vi "Find Control Index in Cluster.vi"(8 "error in (no error)":errorcluster, 10 "Control Name":string, 11 "Cluster ref in":refnum<vi>) -> (0 "error out":errorcluster, 2 "Control Index":i32, 3 "Cluster ref out":refnum<vi>)   [LabVIEW 2019, in "gRPC Template Creation Utility.lvlib"]
uses:
  gRPC Template Creation Utility.lvlib
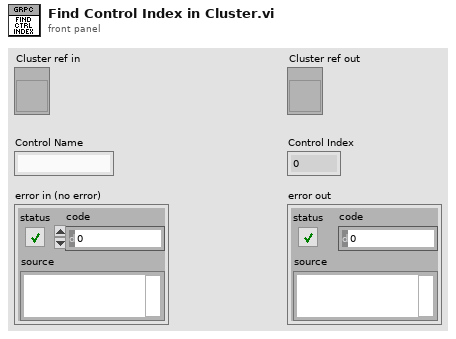
[diagram p1: front panel]
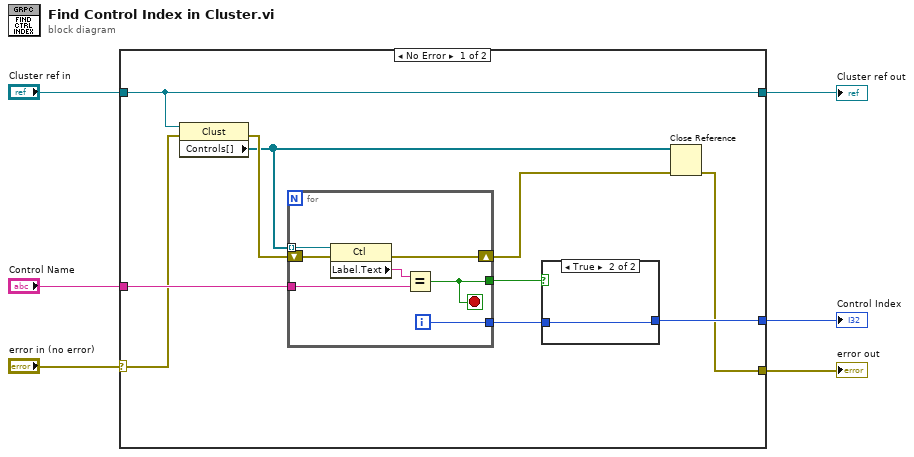
[diagram p0: block diagram]
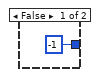
[diagram p2: hidden frame]
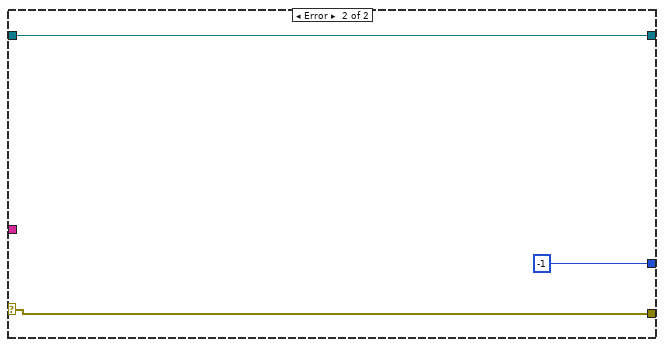
[diagram p3: hidden frame]
diagram:
  n1 = case shown="No Error" "error in (no error)" {
    selector: "error in (no error)" -> [w8 w27]
    tunnel: "Control Name" -> [w11 _]
    tunnel: "Cluster ref in" -> [w7 w26]
    tunnel: [w10 -1] -> w4
    tunnel: [w9 w27] -> w3
    tunnel: [w7 w26] -> w1
    frame No Error {
      n2 = property class="Clust"(reference=w7, error in=w8) -> (error out=w15:errorcluster, "Controls[]"=w14:refnum<vi>[])  [unwired: 1 out]
      n3 = for {
        tunnel: w14 -> [w25] mode=indexing
        tunnel: w11 -> [w24]
        tunnel: [w23] -> w12
        tunnel: [w22] -> w13
        shift-right: [w21] -> w16
        shift-left: w15 -> [w20]
        i -> [w22]
        stop <- w23 stop-if-true
        n4 = property class="Ctl"(reference=w25, error in=w20) -> (error out=w21:errorcluster, "Label.Text"=w19:string)  [unwired: 1 out]
        n5 = Equal?(x=w19, y=w24) -> (x = y?=w23:bool)
      }
      n6 = case shown="True" w12 {
        tunnel: w13 -> [_ w18]
        tunnel: [-1 w18] -> w10
        frame False {
        }
        frame True {
        }
      }
      n7 = Close Reference(reference=w14, error in (no error)=w16) -> (error out=w9:errorcluster)
    }
    frame Error {
    }
  }
  "Control Index" <- w4
  "error out" <- w3
  "Cluster ref out" <- w1
